vi "NATS Open TCP.vi"(6 "timeout ms (5000)":i32=5000, 7 "bytes to read (1024)":i32=1024, 8 "error in":errorcluster, 10 "port (4222)":u16=4222, 11 "address":string="localhost") -> (0 "error out":errorcluster, 1 "server INFO read?":bool, 2 "nats message":T1, 3 "nats connection":T3={"connection ID"=refnum, "server INFO"="", "timeout ms"=25000, "verbose?"=FALSE, "server headers?"=FALSE, "client headers?"=FALSE})   [LabVIEW 2013, in "NATS Core.lvlib"]
doc: "Opens a TCP connection to the NATS server and collects its INFO message."
uses:
  NATS Core.lvlib
  Controls/nats connection.ctl
  Controls/msg type.ctl
  Controls/nats message.ctl
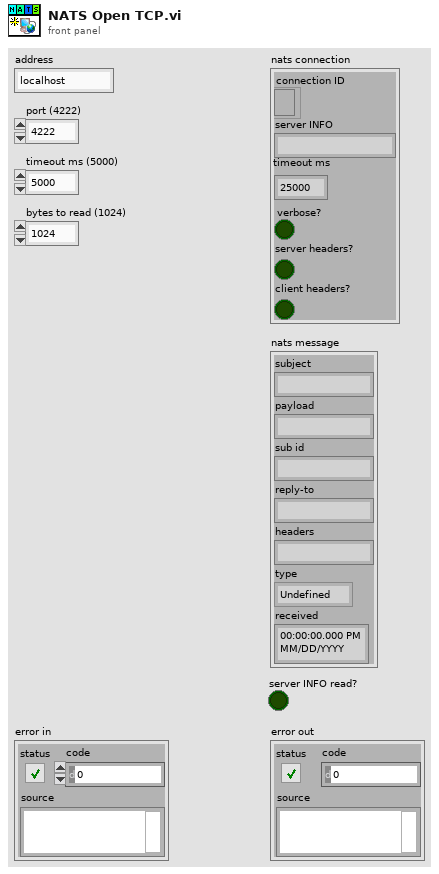
[diagram p1: front panel]
types:
  T1 = typedef "NATS Core.lvlib/nats message.ctl" = cluster{"subject":string, "payload":string, "sub id":string, "reply-to":string, "headers":string, "type":T2, "received":timestamp}
  T2 = typedef "NATS Core.lvlib/msg type.ctl" = enum16{"Undefined", "MSG", "HMSG", "+OK", "PING", "PONG", "-ERR", "INFO"}
  T3 = typedef "NATS Core.lvlib/nats connection.ctl" = cluster{"connection ID":refnum<k5>, "server INFO":string, "timeout ms":i32, "verbose?":bool, "server headers?":bool, "client headers?":bool}
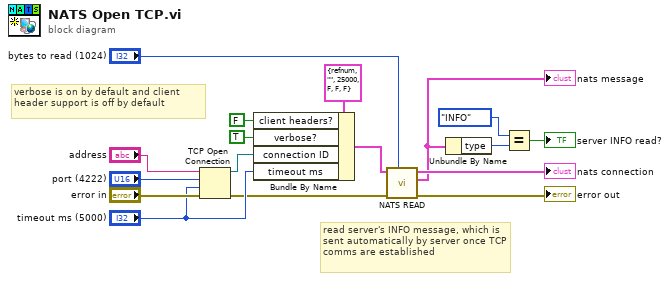
[diagram p0: block diagram]
diagram:
  # "read server's INFO message, which is sent automatically by server once TCP comms are established"
  # "verbose is on by default and client header support is off by default"
  n1 = TCP Open Connection(address="address", remote port or service name="port (4222)", timeout ms (60000)="timeout ms (5000)", error in (no error)="error in") -> (connection ID=w12:refnum<k5>, error out=w10:errorcluster)  [unwired: 1 in]
  n2 = Bundle By Name(cluster=T3 {"connection ID"=refnum, "server INFO"="", "timeout ms"=25000, "verbose?"=FALSE, "server headers?"=FALSE, "client headers?"=FALSE} ("nats connection"), "client headers?"=FALSE, "verbose?"=TRUE, "connection ID"=w12, "timeout ms"="timeout ms (5000)") -> (w9:T3)
  n3 = call "NATS READ.vi"("bytes to read (1024)"="bytes to read (1024)", "error in"=w10, "nats connection in"=w9) -> ("error out"=→"error out":errorcluster, "nats message"=w5:T1, "nats connection out"=→"nats connection":T3)  [unwired: 5 in, 1 out]
  "nats message" <- w5
  n4 = Unbundle By Name(w5) -> ("type"=w4:T2)
  n5 = Equal?(x=msg_type."INFO", y=w4) -> (x = y?=→"server INFO read?":bool)
